vi "CLSUIP_Apply New VI Settings.vi"(5 "Overriding Existing User VI":bool, 7 "Making dynamic?":bool, 8 "error in":errorcluster, 11 "VI in":refnum<vi>) -> (0 "error out":errorcluster, 3 "VI out":refnum<vi>)   [LabVIEW 2021, in "MemberVICreation.lvlib"]
uses:
  <resource>/Framework/Providers/LVClassLibrary/NewAccessors/MemberVICreation.lvlib
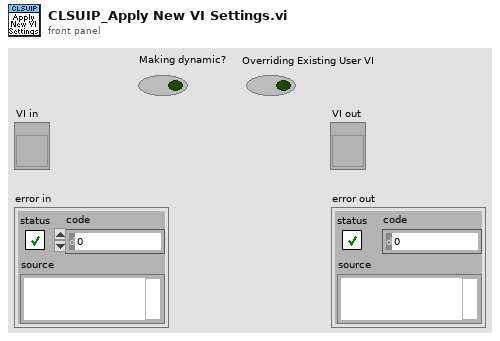
[diagram p1: front panel]
types:
  T1 = enum16{"Share clones between instances", "Preallocate clone for each instance"}
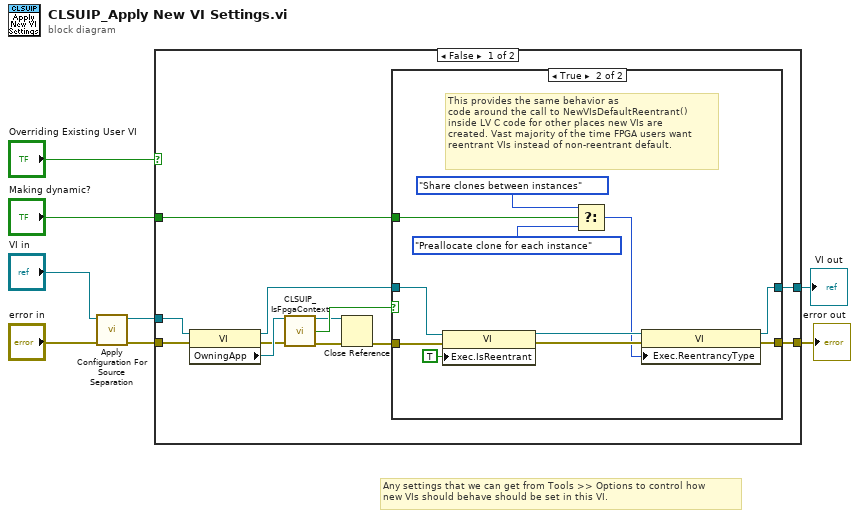
[diagram p0: block diagram]
diagram:
  # "Any settings that we can get from Tools >> Options to control how \nnew VIs should behave should be set in this VI."
  n1 = call <vilib>:"Apply Configuration For Source Separation.vi"("error in (no error)"="error in", "VI in"="VI in") -> ("error out"=w6:errorcluster, "VI out"=w5:refnum<vi>)  [unwired: 8 in]
  n2 = case shown="False" "Overriding Existing User VI" {
    tunnel: w6 -> [w20 w34]
    tunnel: w5 -> [w19 w35]
    tunnel: "Making dynamic?" -> [w11 _]
    tunnel: [w10 w34] -> w3
    tunnel: [w9 w35] -> w2
    frame False {
      n3 = property class="VI"(reference=w19, error in=w20) -> (reference out=w12:refnum<vi>, error out=w17:errorcluster, "OwningApp"=w18:refnum<vi>)
      n4 = call <resource>:"CLSUIP_IsFpgaContext.vi"("context"=w18, "error in (no error)"=w17) -> ("context dup"=w14:refnum<vi>, "is FPGA context"=w16:bool, "error out"=w15:errorcluster)  [unwired: 11 in]
      n5 = Close Reference(reference=w14, error in (no error)=w15) -> (error out=w13:errorcluster)
      n6 = case shown="True" w16 {
        tunnel: w13 -> [w21 w30]
        tunnel: w12 -> [w22 w29]
        tunnel: w11 -> [_ w28]
        tunnel: [w21 w24] -> w10
        tunnel: [w22 w23] -> w9
        frame False {
        }
        frame True {
          # "This provides the same behavior as\ncode around the call to NewVIsDefaultReentrant()\ninside LV C code for other places new VIs are \ncreated. Vast majority of the time FPGA users want \nreentrant VIs instead of non-reentrant default."
          n7 = property class="VI"(reference=w29, error in=w30, "Exec.IsReentrant"=TRUE ("Execution:Is Reentrant")) -> (reference out=w33:refnum<vi>, error out=w32:errorcluster)
          n8 = Select(t=T1."Share clones between instances" ("Execution:Reentrancy Type"), s=w28, f=T1."Preallocate clone for each instance" ("Execution:Reentrancy Type")) -> (s? t:f=w25:T1)
          n9 = property class="VI"(reference=w33, error in=w32, "Exec.ReentrancyType"=w25) -> (reference out=w23:refnum<vi>, error out=w24:errorcluster)
        }
      }
    }
    frame True {
      # "If we are overriding a base class VI,\nwe don't want to override the reentrancy\nsettings. If we did, the VIs would be broken\nbecause the settings wouldn't match."
    }
  }
  "error out" <- w3
  "VI out" <- w2
